vi "Cost.vi"(8 "error in (no error)":errorcluster, 11 "House Blend in":refnum<class "House Blend.lvclass">) -> (0 "error out":errorcluster, 2 "Cost":dbl, 3 "House Blend out":refnum<class "House Blend.lvclass">)   [LabVIEW 2020, in "House Blend.lvclass"]
uses:
  House Blend.lvclass
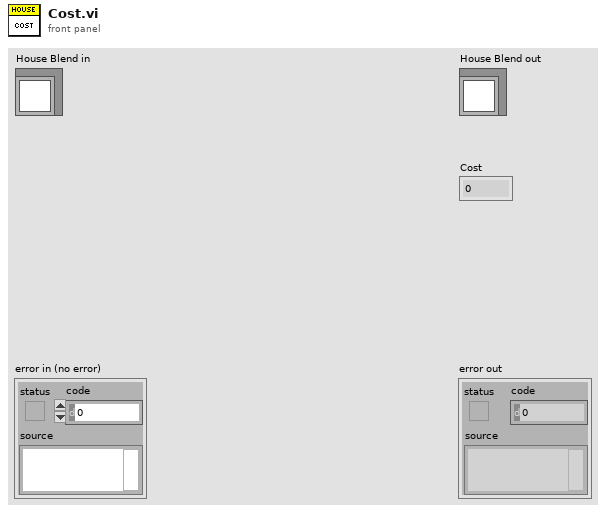
[diagram p1: front panel]
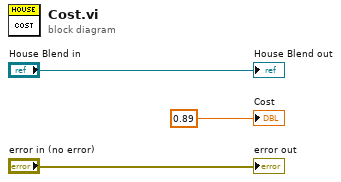
[diagram p0: block diagram]
diagram:
  "error out" <- "error in (no error)"
  "House Blend out" <- "House Blend in"
  "Cost" <- 0.89 ("Cost")
